vi "filterReferee.vi"(6 "Command":string, 8 "error in (no error)":errorcluster, 9 "previous VSS_Ref":T1={"FoulQuadrantVSS"=enum."NO_QUADRANT", "TeamColorVSS"=enum."NONE", "HalfVSS"=enum."SECOND_HALF", "Foul"=enum."GAME_ON", "timestamp"=0.0}, 10 "RefBox UDP RX":T7, 11 "Vision in":refnum<class "Vision.lvclass">) -> (0 "error out":errorcluster, 1 "SSL Referee Game Status":T6 {"Time" format="%<%.3X %x>T"; "Blue Timeout Remaining" format="%<%M:%S>t"; "Yellow Timeout Remaining" format="%<%M:%S>t"; "Time Left" format="%<%M:%S>t"}, 2 "GUI Game Status":T6 {"Time" format="%<%.3X %x>T"; "Blue Timeout Remaining" format="%<%M:%S>t"; "Yellow Timeout Remaining" format="%<%M:%S>t"; "Time Left" format="%<%M:%S>t"}, 3 "Vision out":refnum<class "Vision.lvclass">, 4 "VSS_Ref":T1={"FoulQuadrantVSS"=enum."NO_QUADRANT", "TeamColorVSS"=enum."NONE", "HalfVSS"=enum."SECOND_HALF", "Foul"=enum."FREE_KICK", "timestamp"=0.0}, 5 "RX":bool)   [LabVIEW 2023, in "Vision.lvclass"]
uses:
  Vision.lvclass
  Controls/vision_control.ctl
  Old vision/Decode SSL and Refree Wrapper Package Folder/SSL Referee Game Status.ctl
  Referee_class/VSS_Ref.ctl
  Referee_class/Quadrant.ctl
  Referee_class/Color.ctl
  Referee_class/Halfs.ctl
  Referee_class/commands.ctl
  Referee_class/Referee.lvclass
panel:
  # "Score"
  # "Red Cards"
  # "Yellow Cards"
  # "Timeouts Left"
  # "Timeout Remaining"
  # "Goalie ID"
  # "Score"
  # "Red Cards"
  # "Yellow Cards"
  # "Timeouts Left"
  # "Timeout Remaining"
  # "Goalie ID"
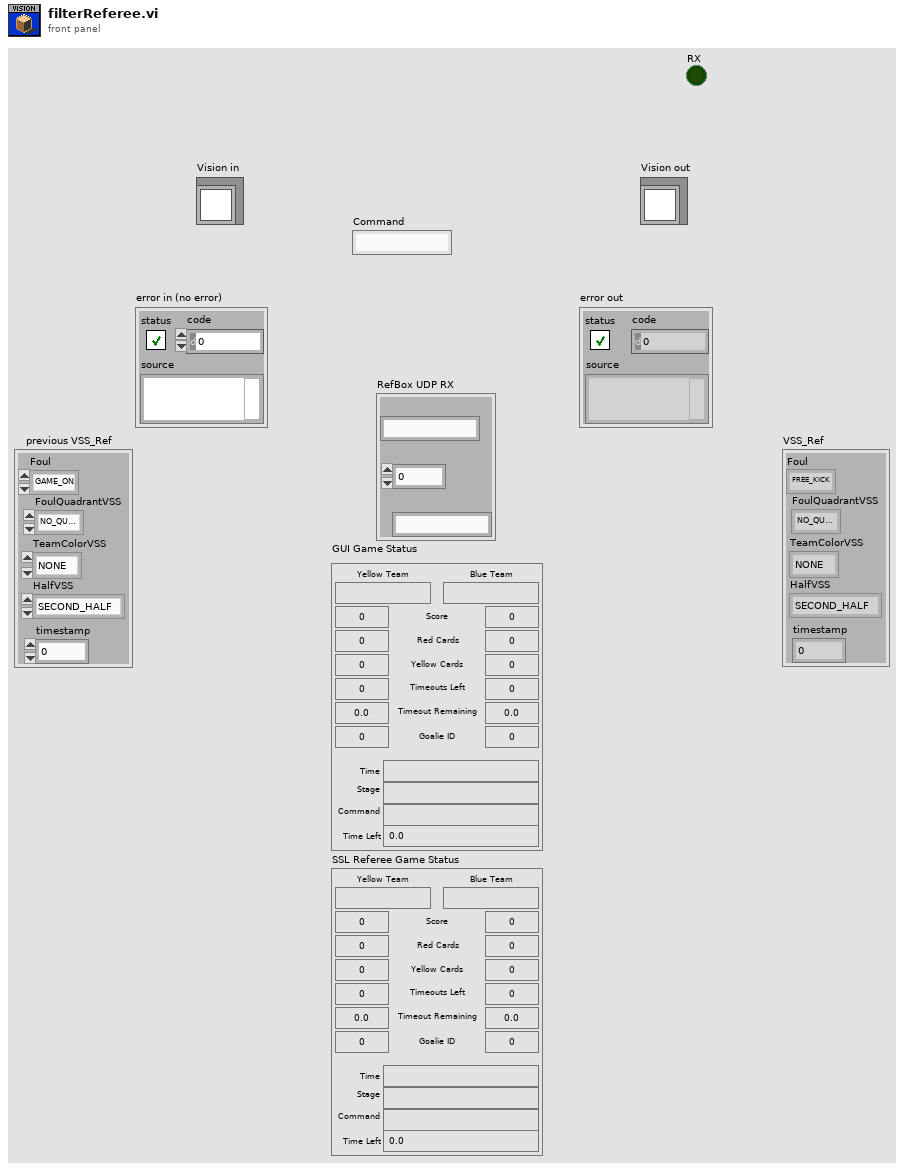
[diagram p1: front panel]
types:
  T1 = typedef "Referee.lvclass/VSS_Ref.ctl" = cluster{"FoulQuadrantVSS":T2, "TeamColorVSS":T3, "HalfVSS":T4, "Foul":T5, "timestamp":dbl}
  T2 = typedef "Quadrant.ctl" = enum16{"NO_QUADRANT", "QUADRANT_1", "QUADRANT_2", "QUADRANT_3", "QUADRANT_4"}
  T3 = typedef "Color.ctl" = enum16{"BLUE", "YELLOW", "NONE"}
  T4 = typedef "Halfs.ctl" = enum16{"NO_HALF", "FIRST_HALF", "SECOND_HALF", "OVERTIME_FIRST_HALF", "OVERTIME_SECOND_HALF", "PENALTY_SHOOTOUS"}
  T5 = typedef "Referee.lvclass/commands.ctl" = enum16{"FREE_KICK", "PENALTY_KICK", "GOAL_KICK", "FREE_BALL", "KICKOFF", "STOP", "GAME_ON", "HALT"}
  T6 = typedef "SSL Referee Game Status.ctl" = cluster{"Stage":string, "Command":string, "Time Left":dbl, "Yellow Team":string, "Blue Team":string, "Yellow Score":u32, "Blue Score":u32, "Yellow Red Cards":u32, "Blue Red Cards":u32, "Yellow Yellow Cards":u32, "Blue Yellow Cards":u32, "Yellow Timeouts Left":u32, "Blue Timeouts Left":u32, "Yellow Timeout Remaining":dbl, "Blue Timeout Remaining":dbl, "Yellow Goalie Id":u32, "Blue Goalie Id":u32, "Time":timestamp}
  T7 = typedef "vision_control.ctl" = cluster{"Local IP:":string, "Port":i32, "Server IP:":string}
  T8 = typedef "SSL Referee.ctl" = cluster{"packet_\ntimestamp":u64, "stage":u64, "stage_time_left":i32, "command ":u64, "command_\ncounter ":u32, "command_\ntimestamp":u64, "yellow team info":T9, "blue team info":T9, "Point":cluster{"x":sgl, "y":sgl}}
  T9 = typedef "SSL Referee Team Info.ctl" = cluster{"name":string, "score":u32, "red_cards":u32, "yellow_cards_time":u32[], "yellow_cards":u32, "timeout":u32, "timeout_times":u32, "goalie":u32}
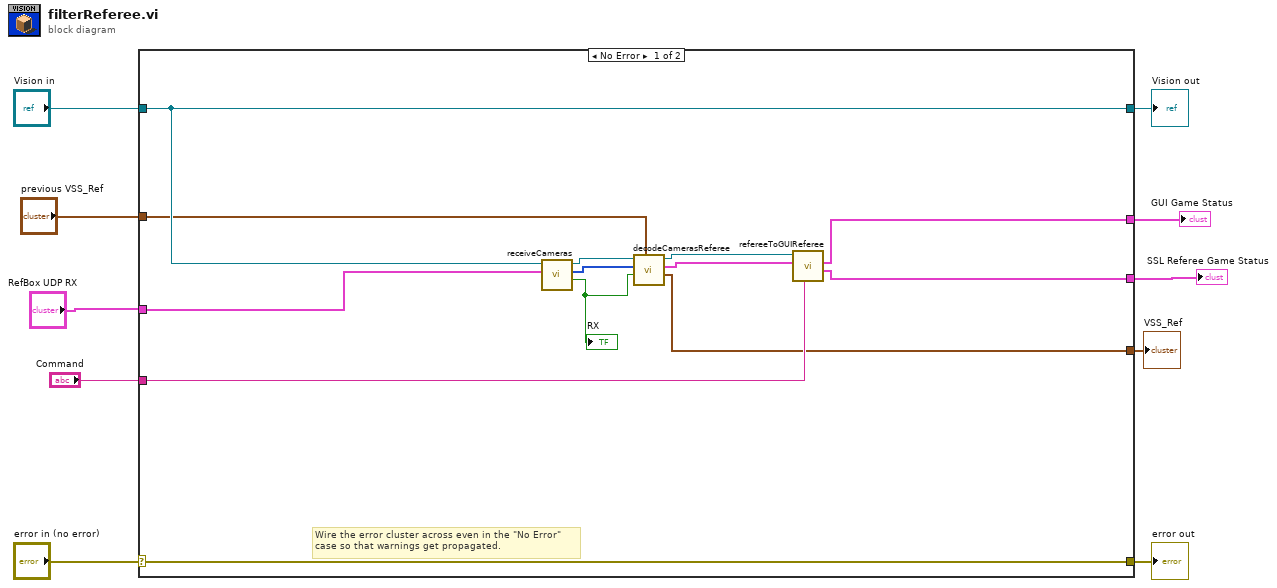
[diagram p0: block diagram]
diagram:
  n1 = case shown="No Error" "error in (no error)" {
    selector: "error in (no error)" -> [w23 w25]
    tunnel: [w23 w25] -> w9
    tunnel: [w17 w24] -> w7
    tunnel: "Vision in" -> [w17 w24]
    tunnel: "RefBox UDP RX" -> [w18 _]
    tunnel: [w16 _] -> w5
    tunnel: [w15 _] -> w4
    tunnel: "Command" -> [w14 _]
    tunnel: [w13 _] -> w1
    tunnel: "previous VSS_Ref" -> [w11 _]
    frame No Error {
      # "Wire the error cluster across even in the \"No Error\"\ncase so that warnings get propagated."
      n2 = call "receiveCameras.vi"("Cluster"=w18, "Vision in"=w17) -> ("RX"=w12:bool, "data camera out"=w21:u8[], "Vision out"=w19:refnum<class "Vision.lvclass">)  [unwired: 5 in, 1 out]
      "RX" <- w12
      n3 = call "decodeCamerasReferee.vi"("previous VSS_Ref"=w11, "RX"=w12, "element"=w21, "Vision in"=w19) -> ("VSS_Ref"=w13:T1, "SSL Game Status"=w22:T8, "Vision out"=w20:refnum<class "Vision.lvclass">)  [unwired: 4 in, 1 out]
      n4 = call "refereeToGUIReferee.vi"("Command"=w14, "SSL Game Status"=w22, "Vision in"=w20) -> ("SSL Referee Game Status"=w15:T6, "GUI Game Status"=w16:T6)  [unwired: 5 in, 2 out]
    }
    frame Error {
    }
  }
  "error out" <- w9
  "Vision out" <- w7
  "GUI Game Status" <- w5
  "SSL Referee Game Status" <- w4
  "VSS_Ref" <- w1
